vi "c_ctre_phoenix6_SetUpdateFrequencyForAll.vi"(0 "Numeric 2":i32, 1 "Cluster":T1, 2 "Numeric 3":u32, 3 "Numeric 4":dbl, 4 "Numeric 5":dbl) -> (20 "Numeric":i32)   [LabVIEW 2023]
uses:
  <vilib>/Rock Robotics/WPI/ThirdParty/Phoenix-LabVIEW/Controls/DriverLib.ctl
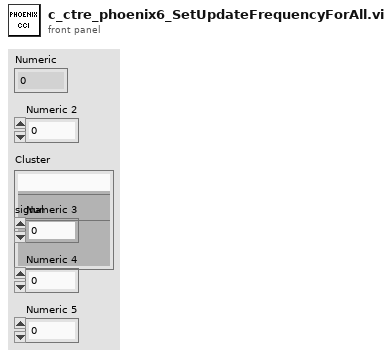
[diagram p1: front panel]
types:
  T1 = cluster{"Network":string, "signal":cluster{"deviceHash":u32, "spn":u32}}
  T2 = typedef "DriverLib.ctl" = path
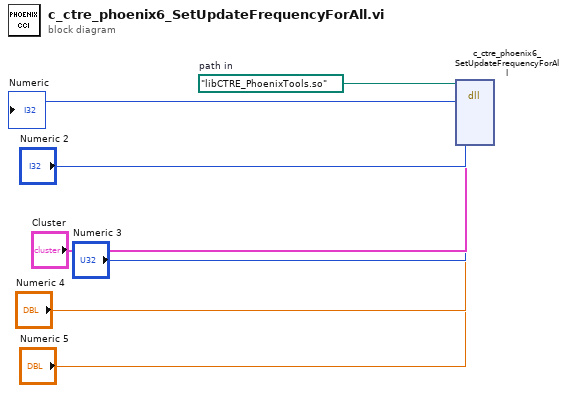
[diagram p0: block diagram]
diagram:
  w7 = T2 path "libCTRE_PhoenixTools.so"  # path in
  n1 = dll-call lib="?" fn="c_ctre_phoenix6_SetUpdateFrequencyForAll"(path in=w7, "Numeric 2", "Cluster", "Numeric 3", "Numeric 4", "Numeric 5") -> (→"Numeric":i32)  [unwired: 7 in, 2 out]
